vi "ManualUpload.vi"() -> ()   [LabVIEW 2020]
uses:
  Keithley_Subs/CapacitanceInfos.ctl
  Keithley_Subs/CapacitanceRecord.ctl
  <vilib>/Utility/file.llb/Read Delimited Spreadsheet (DBL).vi
  <vilib>/httpClient/POSTBuffer.vi
  <vilib>/httpClient/LabVIEWHTTPClient.lvlib
panel:
  out "array":string[][](array[string])
  out "All Files in Dir":path[](array[path])
  in  "SideLength":dbl=1.0
  in  "Area":dbl=1.0
  in  "Cluster 3":T3={"Intercept Error"=0.0, "Slope Error"=0.0, "Intercept"=0.0, "Slope"=0.0, "DataType"="", "Current"=[], "Voltage"=[], "Capacitance"=0.0, "Area"=0.0, "SideLength"=0.0, "InfoCluster"={"Conductance"=0.0, "CapacitanceIV"=0.0, "Intercept"=0.0, "CapacitanceSW"=0.0, "Sum"=0.0, "CapacitanceInfos"=[], "CapacitancePhase"=0.0, "dC/dV"=0.0, "Function"="", "OtherInfo"=[]}, "TimeStep"=0.0, "Source"="ProbeStation", "Title"="", "experimentDate"=""}
  out "error out":errorcluster
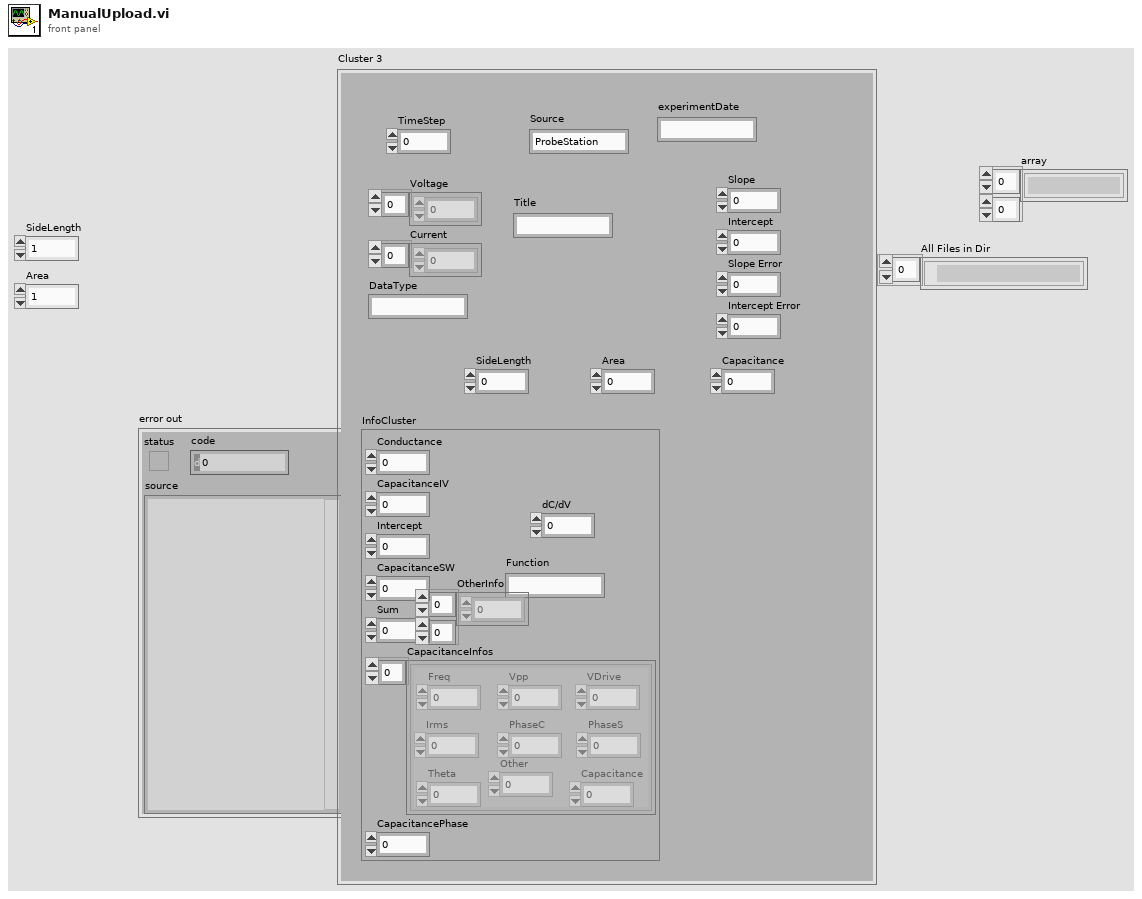
[diagram p1: front panel]
types:
  T1 = typedef "CapacitanceInfos.ctl" = cluster{"Conductance":dbl, "CapacitanceIV":dbl, "Intercept":dbl, "CapacitanceSW":dbl, "Sum":dbl, "CapacitanceInfos":T2[], "CapacitancePhase":dbl, "dC/dV":dbl, "Function":string, "OtherInfo":dbl[][]}
  T2 = typedef "CapacitanceRecord.ctl" = cluster{"Freq":dbl, "Vpp":dbl, "PhaseS":dbl, "Irms":dbl, "PhaseC":dbl, "Theta":dbl, "VDrive":dbl, "Capacitance":dbl, "Other":dbl}
  T3 = cluster{"Intercept Error":dbl, "Slope Error":dbl, "Intercept":dbl, "Slope":dbl, "DataType":string, "Current":dbl[], "Voltage":dbl[], "Capacitance":dbl, "Area":dbl, "SideLength":dbl, "InfoCluster":T1, "TimeStep":dbl, "Source":string, "Title":string, "experimentDate":string}
  T4 = typedef "LabVIEWHTTPClient.lvlib/ClientHandle.ctl" = refnum<k1>
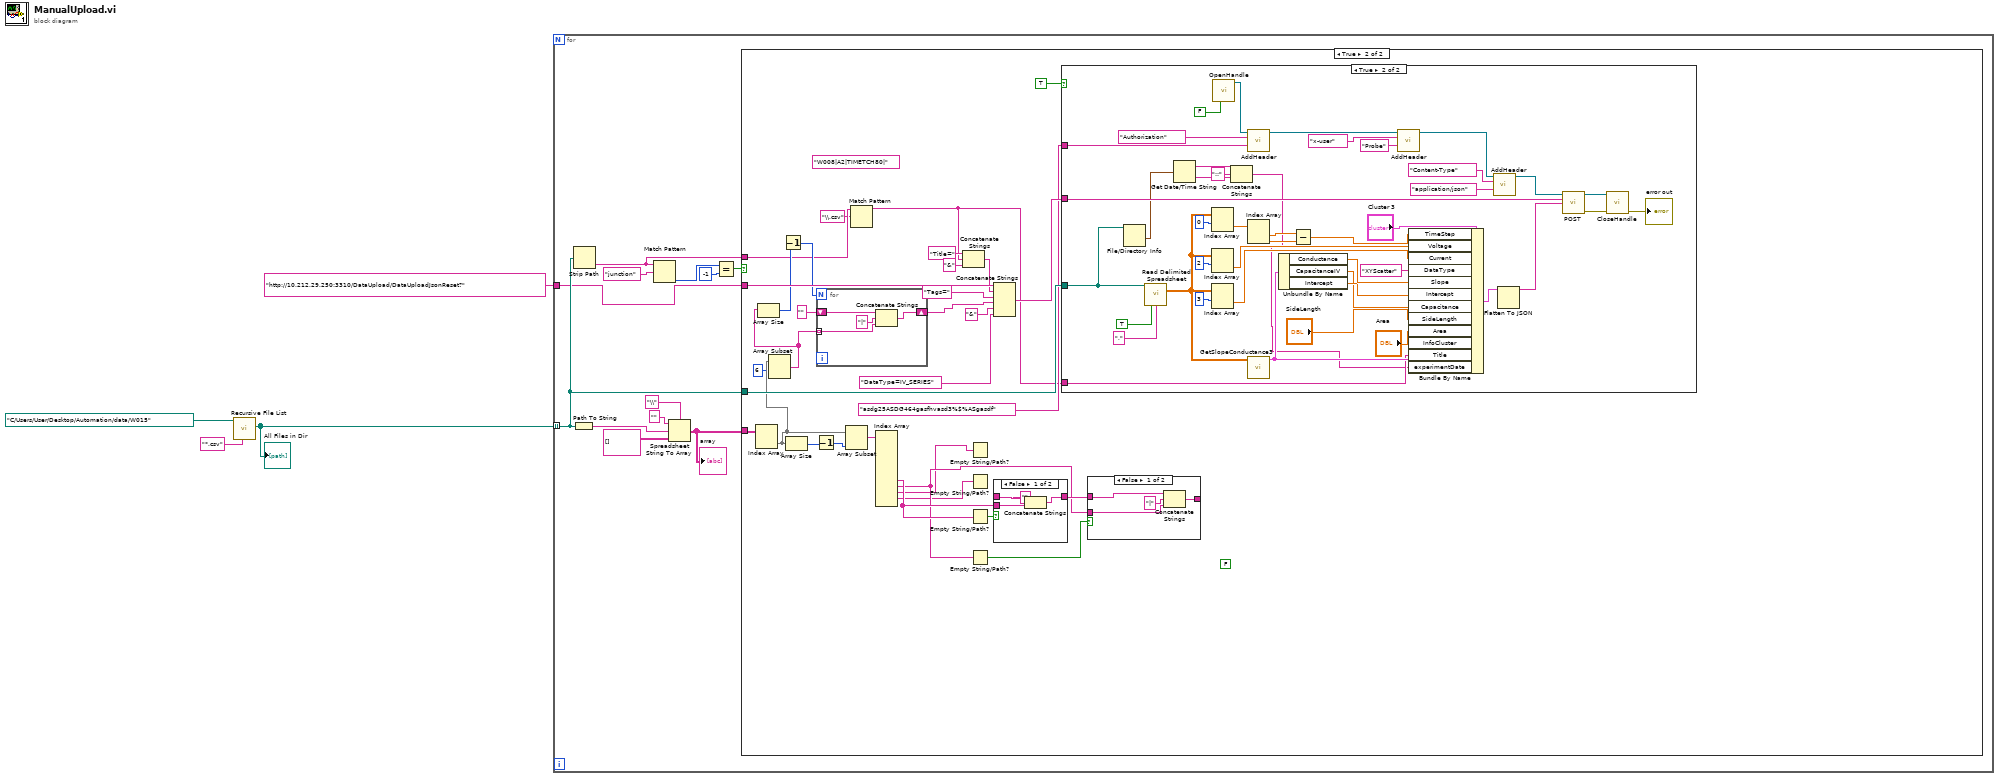
[diagram p0: block diagram]
diagram:
  n1 = call <vilib>:"Recursive File List.vi"("pattern"="*.csv", "Folder Path"=path "C:/Users/User/Desktop/Automation/data/W015" ("path")) -> ("All Files in Dir"=w2:path[])  [unwired: 5 in, 4 out]
  "All Files in Dir" <- w2
  n2 = for {
    tunnel: w2 -> [w14] mode=indexing
    tunnel: "http://10.212.29.250:3310/DataUpload/DataUploadJsonReset?" ("input string") -> [w5]
    n3 = Path To String(path=w14) -> (string=w13:string)
    n4 = Strip Path(path=w14) -> (name=w16:string)  [unwired: 1 out]
    n5 = Match Pattern(string=w16, regular expression="junction") -> (offset past match=w9:i32)  [unwired: 1 in, 3 out]
    n6 = Spreadsheet String To Array(delimiter (Tab)="\\" ("search string/char (-)"), format string="", spreadsheet string=w13, array type (2D Dbl)=string[][] []) -> (array=w6:string[][])
    "array" <- w6
    n7 = Equal?(x=w9, y=-1) -> (x = y?=w7:bool)
    n8 = case shown="True" w7 {
      tunnel: w16 -> [_ w22]
      tunnel: w14 -> [_ w49]
      tunnel: w5 -> [_ w48]
      tunnel: w6 -> [_ w42]
      frame False {
      }
      frame True {
        (unwired) "W008|A2|TIMETCH80|"
        (unwired) FALSE
        n9 = Index Array(array=w42) -> (element=w28:string[])  [unwired: 2 in]
        n10 = Array Subset(array=w28, index=6) -> (w25:string[])  [unwired: 1 in]
        n11 = Array Size(array=w25) -> (size(s)=w24:i32)
        n12 = Decrement(x=w24) -> (x-1=w23:i32)
        n13 = Array Size(array=w28) -> (size(s)=w34:i32)
        n14 = Decrement(x=w34) -> (x-1=w33:i32)
        n15 = for {
          N: w23 -> [_]
          shift-right: [w105] -> w26
          shift-left: "" -> [w104]
          tunnel: w25 -> [w103] mode=indexing
          n16 = Concatenate Strings(w104, "|" ("string"), w103) -> (w105:string)
        }
        n17 = Array Subset(array=w28, length=w33) -> (w35:string[])  [unwired: 1 in]
        n18 = Match Pattern(string=w22, regular expression="\\.csv") -> (before substring=w19:string)  [unwired: 1 in, 3 out]
        n19 = Index Array(array=w35) -> (element #7=w32:string, element #8=w31:string, element #9=w30:string, element #10=w29:string)  [unwired: 11 in, 7 out]
        n20 = Concatenate Strings("Title=" ("string"), w19, "&" ("string")) -> (w18:string)
        n21 = Empty String/Path?(string/path=w30) -> ()  [unwired: 1 out]
        n22 = Empty String/Path?(string/path=w29) -> ()  [unwired: 1 out]
        n23 = Empty String/Path?(string/path=w32) -> (empty?=w40:bool)
        n24 = Empty String/Path?(string/path=w31) -> (empty?=w39:bool)
        n25 = Concatenate Strings(w48, w18, "Tags=" ("string"), w26, "&" ("string"), "DataType=IV_SERIES" ("string")) -> (w46:string)
        n26 = case shown="False" w40 {
          tunnel: "" -> [w101 w102]
          tunnel: [w100 w102] -> w38
          tunnel: w32 -> [w99 _]
          frame False {
            n27 = Concatenate Strings(w101, w99) -> (w100:string)
          }
          frame True {
          }
        }
        n28 = case shown="True" TRUE {
          tunnel: w49 -> [_ w55]
          tunnel: w46 -> [_ w63]
          tunnel: "asdg25ASDG464gasfhvasd3%$%ASgasdf" ("value") -> [_ w57]
          tunnel: w19 -> [_ w56]
          frame False {
          }
          frame True {
            n29 = File/Directory Info(path=w55) -> (last mod=w54:timestamp)  [unwired: 1 in, 6 out]
            n30 = call-poly <vilib>:"Read Delimited Spreadsheet.vi"("file path (dialog if empty)"=w55, "transpose? (F)"=TRUE, "delimiter (\\t)"="," ("delimiter (\\t)")) -> ("all rows"=w71:dbl[][])  [unwired: 7 in, 5 out]
            n31 = Get Date/Time String(seconds (now)=w54) -> (date string=w53:string, time string=w52:string)  [unwired: 2 in]
            n32 = Index Array(array=w71, index (row)=0) -> (element=w68:dbl[])  [unwired: 1 in]
            n33 = Index Array(array=w71, index (row)=2) -> (element=w90:dbl[])  [unwired: 1 in]
            n34 = Index Array(array=w71, index (row)=3) -> (element=w91:dbl[])  [unwired: 1 in]
            n35 = call <vilib>:"OpenHandle.vi"("verify server(true)"=FALSE) -> ("client handle out"=w58:T4)  [unwired: 13 in, 1 out]
            n36 = Concatenate Strings(w53, "::" ("string"), w52) -> (w50:string)
            n37 = call <vilib>:"AddHeader.vi"("client handle"=w58, "header"="Authorization", "value"=w57) -> ("client handle out"=w82:T4)  [unwired: 11 in, 1 out]
            n38 = Index Array(array=w68) -> (element #1=w66:dbl, element #2=w67:dbl)  [unwired: 2 in]
            n39 = call "GetSlopeConductance3.vi"("Array in"=w71) -> ("InfoCluster"=w70:T1)  [unwired: 9 in, 1 out]
            n40 = Unbundle By Name(w70) -> ("Conductance"=w78:dbl, "CapacitanceIV"=w76:dbl, "Intercept"=w77:dbl)
            n41 = Subtract(x=w66, y=w67) -> (x-y=w65:dbl)
            n42 = call <vilib>:"AddHeader.vi"("client handle"=w82, "header"="x-user", "value"="Probe") -> ("client handle out"=w73:T4)  [unwired: 11 in, 1 out]
            n43 = Bundle By Name(cluster="Cluster 3", "TimeStep"=w65, "Voltage"=w90, "Current"=w91, "DataType"="XYScatter", "Slope"=w78, "Intercept"=w77, "Capacitance"=w76, "SideLength"="SideLength", "Area"="Area", "InfoCluster"=w70, "Title"=w56, "experimentDate"=w50) -> (w93:T3)
            n44 = call <vilib>:"AddHeader.vi"("client handle"=w73, "header"="Content-Type", "value"="application/json") -> ("client handle out"=w72:T4)  [unwired: 11 in, 1 out]
            n45 = Flatten To JSON(anything=w93) -> (JSON string=w86:string)  [unwired: 2 in, 1 out]
            n46 = call-poly <vilib>:"POST.vi"("client handle"=w72, "url"=w63, "buffer"=w86) -> ("client handle out"=w60:T4, "error out"=w59:errorcluster)  [unwired: 9 in, 2 out]
            n47 = call <vilib>:"CloseHandle.vi"("client handle"=w60, "error in (no error)"=w59) -> ("error out"=→"error out":errorcluster)  [unwired: 13 in]
          }
        }
        n48 = case shown="False" w39 {
          tunnel: w38 -> [w97 w98]
          tunnel: [w96 w98] -> _
          tunnel: w31 -> [w94 _]
          frame False {
            n49 = Concatenate Strings(w97, "|" ("string"), w94) -> (w96:string)
          }
          frame True {
          }
        }
      }
    }
  }
